vi "Generate a static LineScan Image.vi"(7 "Generate Static Image Options":T1(ring), 8 "error in (no error)":errorcluster) -> (0 "error out":errorcluster)   [LabVIEW 2012]
doc: "SciScan 1.2 160622"
uses:
  GFG/GFGnumericGet.vi
  GFG/GFGImageRefsGet.vi
  GFG/GFG library.lvlib
panel:
  out "y.pixels":dbl
  out "nomin.x.pixels":dbl
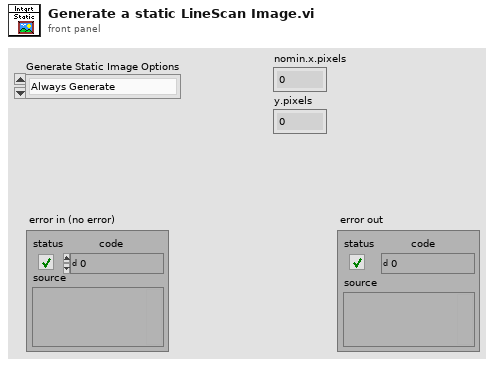
[diagram p1: front panel]
types:
  T1 = enum16{"Always Generate", "Generate if no valid image"}
  T2 = cluster{"xyvoltagefor2frames":dbl[][][], "x.pixels":dbl, "nomin.x.pixels":dbl, "y.pixels":dbl, "fill.fraction":dbl, "x.bidirectional":bool, "y.bidirectional":bool}
  T3 = typedef "IMAQ Image.ctl" = refnum<image>
  T4 = cluster{"Channel 1 small":T3, "Channel 2 small":T3, "Channel 3 small":T3, "Channel 4 small":T3, "Channel 1 large":T3, "Channel 2 large":T3, "Channel 3 large":T3, "Channel 4 large":T3, "RGB overlay":T3, "ROI Image display":T3, "arb line scan display":T3, "Channel 5 large":T3}
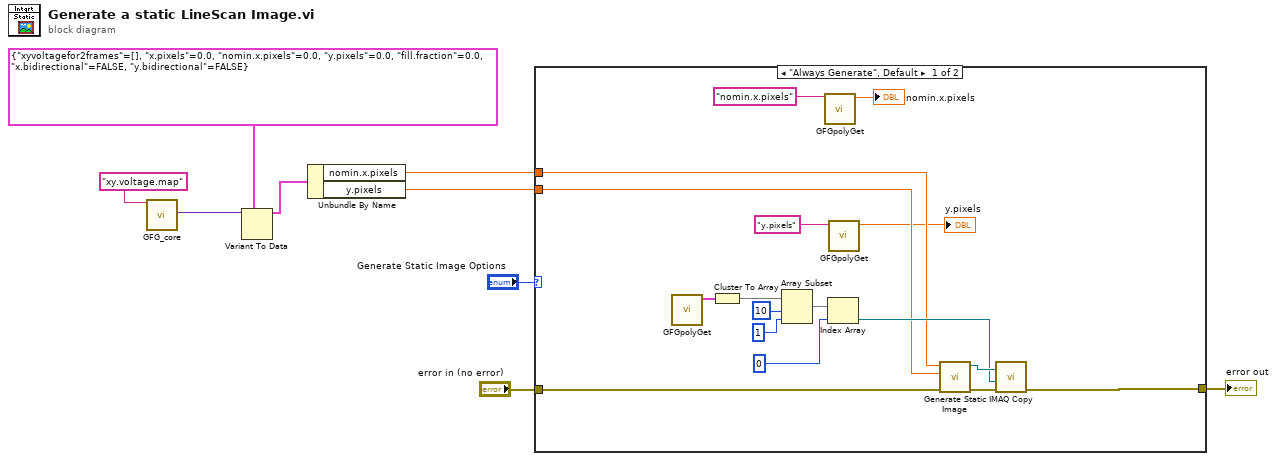
[diagram p0: block diagram]
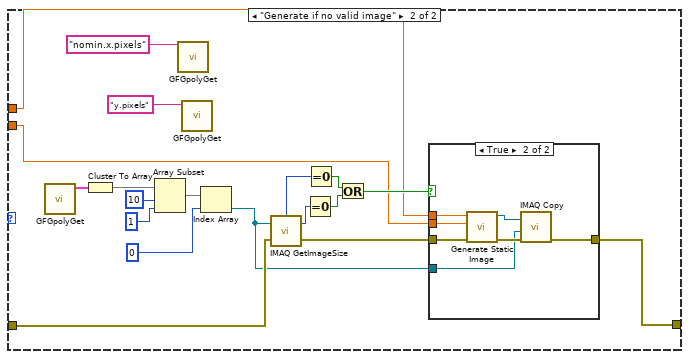
[diagram p2: hidden frame]
diagram:
  n1 = call "GFG_core.vi"("Variable Name in"="xy.voltage.map") -> ("Variant Out"=w5:variant)  [unwired: 12 in, 6 out]
  n2 = Variant To Data(type=T2 {"xyvoltagefor2frames"=[], "x.pixels"=0.0, "nomin.x.pixels"=0.0, "y.pixels"=0.0, "fill.fraction"=0.0, "x.bidirectional"=FALSE, "y.bidirectional"=FALSE} ("output cluster"), Variant=w5) -> (data=w3:T2)  [unwired: 1 in, 1 out]
  n3 = Unbundle By Name(w3) -> ("nomin.x.pixels"=w2:dbl, "y.pixels"=w1:dbl)
  n4 = case shown="\"Always Generate\", Default" "Generate Static Image Options" {
    tunnel: "error in (no error)" -> [w15 w33]
    tunnel: [w14 w29] -> w8
    tunnel: w2 -> [w13 w28]
    tunnel: w1 -> [w12 w27]
    frame "Always Generate", Default {
      n5 = call-poly "GFGpolyGet.vi"() -> ("Image Refs Out"=w21:T4)  [unwired: 10 in, 1 out]
      n6 = Cluster To Array(cluster=w21) -> (array=w20:T3[])
      n7 = Array Subset(array=w20, index=10, length=1) -> (w18:T3[])
      n8 = call-poly "GFGpolyGet.vi"("Variable Name in"="nomin.x.pixels") -> ("Numeric"=→"nomin.x.pixels":dbl)  [unwired: 8 in, 2 out]
      n9 = Index Array(array=w18, index=0) -> (element=w16:T3)
      n10 = call-poly "GFGpolyGet.vi"("Variable Name in"="y.pixels" ("Tag in")) -> ("Numeric"=→"y.pixels":dbl)  [unwired: 8 in, 2 out]
      n11 = call "Generate Static Image.vi"("error in (no error)"=w15, "Image Y Size"=w12, "Image X Size"=w13) -> ("error out"=w25:errorcluster, "Image 2"=w26:T3)  [unwired: 7 in]
      n12 = call "IMAQ Copy"("error in (no error)"=w25, "Image Dst"=w16, "Image Src"=w26) -> ("error out"=w14:errorcluster)  [unwired: 3 in, 1 out]
    }
    frame "Generate if no valid image" {
      n13 = call-poly "GFGpolyGet.vi"() -> ("Image Refs Out"=w42:T4)  [unwired: 10 in, 1 out]
      n14 = Cluster To Array(cluster=w42) -> (array=w41:T3[])
      n15 = Array Subset(array=w41, index=10, length=1) -> (w39:T3[])
      n16 = call-poly "GFGpolyGet.vi"("Variable Name in"="nomin.x.pixels") -> ()  [unwired: 8 in, 3 out]
      n17 = call-poly "GFGpolyGet.vi"("Variable Name in"="y.pixels" ("Tag in")) -> ()  [unwired: 8 in, 3 out]
      n18 = Index Array(array=w39, index=0) -> (element=w30:T3)
      n19 = call "IMAQ GetImageSize"("Image"=w30, "error in (no error)"=w33) -> ("Y Resolution"=w36:i32, "X Resolution"=w37:i32, "error out"=w31:errorcluster)  [unwired: 2 in]
      n20 = Equal To 0?(x=w36) -> (x = 0?=w35:bool)
      n21 = Equal To 0?(x=w37) -> (x = 0?=w34:bool)
      n22 = Or(x=w34, y=w35) -> (x .or. y?=w32:bool)
      n23 = case shown="True" w32 {
        tunnel: w28 -> [_ w53]
        tunnel: w27 -> [_ w52]
        tunnel: w31 -> [w46 w51]
        tunnel: w30 -> [_ w48]
        tunnel: [w46 w47] -> w29
        frame False {
        }
        frame True {
          n24 = call "Generate Static Image.vi"("error in (no error)"=w51, "Image Y Size"=w52, "Image X Size"=w53) -> ("error out"=w50:errorcluster, "Image 2"=w49:T3)  [unwired: 7 in]
          n25 = call "IMAQ Copy"("error in (no error)"=w50, "Image Dst"=w48, "Image Src"=w49) -> ("error out"=w47:errorcluster)  [unwired: 3 in, 1 out]
        }
      }
    }
  }
  "error out" <- w8
